vi "Model - Get DB Records2 Array.vi"(8 "error in (no error)":errorcluster, 11 "View Model":T4) -> (0 "error out":errorcluster, 2 "DB Record2 Array":T1[](array[typedef]), 3 "View Model":T4)   [LabVIEW 2017]
doc: "Get actual value of DB Records 2 Array from DVR"
uses:
  Controls/View Model.ctl
  Controls/Shared Model.ctl
  Error Handler/Controls/Error Model.ctl
  Error Handler/Controls/Error Message.ctl
  Error Handler/Controls/Error Type.ctl
  Configuration/Controls/Config Model.ctl
  Configuration/Controls/Config DB Message.ctl
  Configuration/Controls/Config DB Command.ctl
  Configuration/Controls/Config DB Overhead.ctl
  Configuration/Controls/Config DB Record1.ctl
  Configuration/Controls/Config DB Record2.ctl
  Controller/Controls/Controller Wash Step.ctl
  Views/Vehicle Position Simulation View/Controls/Vehicle - Position.ctl
  Controller/Controls/Controller Model.ctl
  Controller/Controls/Controller Overhead.ctl
  Controller/Controls/Controller State.ctl
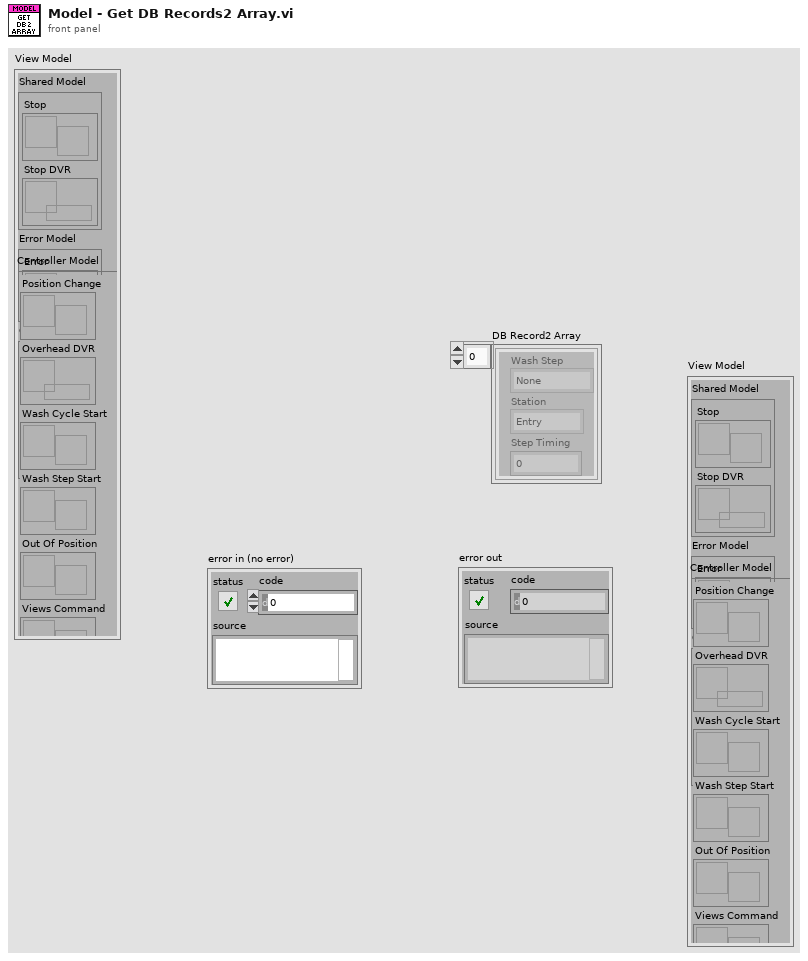
[diagram p1: front panel]
types:
  T1 = typedef "Config DB Record2.ctl" = cluster{"Wash Step":T2, "Station":T3, "Step Timing":u32}
  T2 = typedef "Controller Wash Step.ctl" = enum16{"None", "Under Body Wash", "Bug Remover", "Pre-Soak", "High Pressure Wash", "Low Pressure Wax", "Spot Free Rinse", "Tire Shine Foam", "Air Dry"}
  T3 = typedef "Vehicle - Position.ctl" = enum16{"Entry", "Station 1", "Station 2", "Station 3", "Exit"}
  T4 = typedef "View Model.ctl" = cluster{"Shared Model":T5, "Error Model":T6, "Config Model":T7, "Controller Model":T8}
  T5 = typedef "Shared Model.ctl" = cluster{"Stop":refnum<user-event>, "Stop DVR":refnum<data-value>}
  T6 = typedef "Error Model.ctl" = cluster{"Error":refnum<user-event>}
  T7 = typedef "Config Model.ctl" = cluster{"Config":refnum<user-event>, "Config DVR":refnum<data-value>}
  T8 = typedef "Controller Model.ctl" = cluster{"Position Change":refnum<user-event>, "Overhead DVR":refnum<data-value>, "Wash Cycle Start":refnum<user-event>, "Wash Step Start":refnum<user-event>, "Out Of Position":refnum<user-event>, "Views Command":refnum<user-event>}
  T9 = typedef "Config DB Overhead.ctl" = cluster{"Locked DB?":bool, "DB Record1 Array":T10[], "Queried Step Duration":u32, "DB Record2 Array":T1[]}
  T10 = typedef "Config DB Record1.ctl" = cluster{"Wash Step":string, "Station":string, "Step Duration":u32}
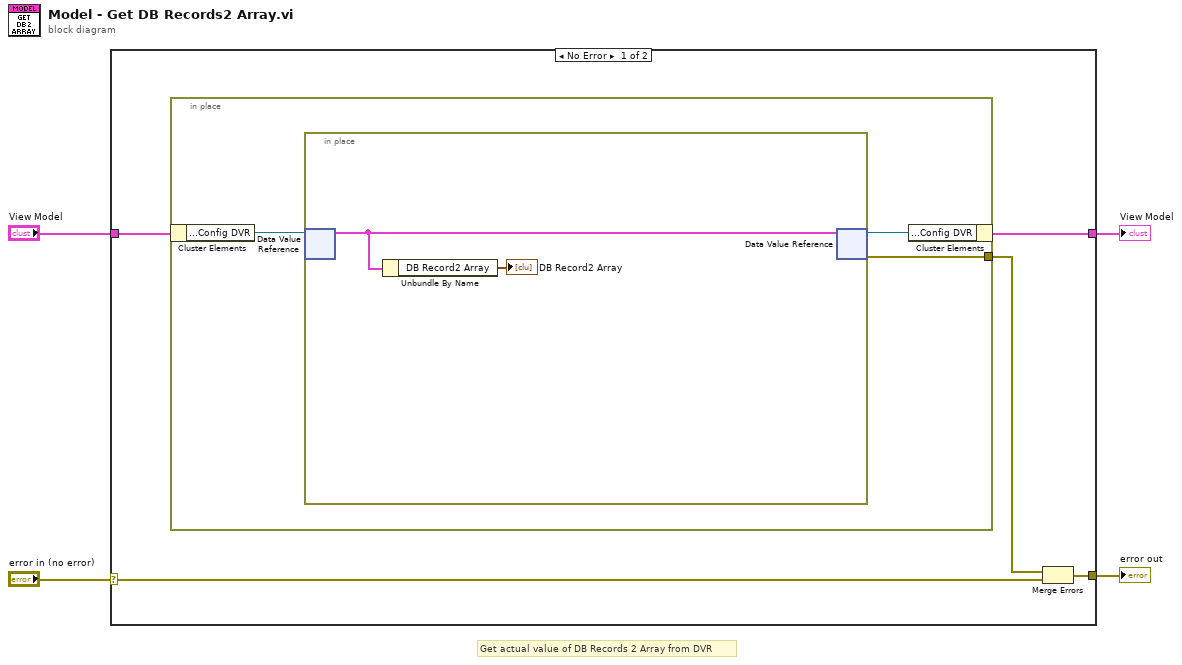
[diagram p0: block diagram]
diagram:
  # "Get actual value of DB Records 2 Array from DVR"
  n1 = case shown="No Error" "error in (no error)" {
    selector: "error in (no error)" -> [w7 w16]
    tunnel: "View Model" -> [w9 w15]
    tunnel: [w6 w16] -> w2
    tunnel: [w5 w15] -> w1
    frame No Error {
      n2 = in-place {
        in-place-border: [w10] -> w8
        n3 = in-place-cluster #1(w9) -> ("Config Model.Config DVR"=w12:refnum<data-value>)
        n4 = in-place {
          n5 = in-place-dvr #2(w12) -> (w14:T9)  [unwired: 1 out]
          n6 = Unbundle By Name(w14) -> ("DB Record2 Array"=→"DB Record2 Array":T1[])
          n7 = in-place-dvr #2(w14) -> (w11:refnum<data-value>, w10:errorcluster)
        }
        n8 = in-place-cluster #1("Config Model.Config DVR"=w11) -> (w5:T4)
      }
      n9 = Merge Errors(w8, w7) -> (w6:errorcluster)
    }
    frame Error {
    }
  }
  "View Model" <- w1
  "error out" <- w2
